vi "mqttCmdPublishCreate.vi"(6 "connMeta":T1, 8 "error in (no error)":errorcluster, 9 "value":string, 10 "topic":string) -> (0 "error out":errorcluster, 3 "mqttCmdPublish out":refnum<class "PublishMqttMsg.lvclass">)   [LabVIEW 2020, in "PublishMqttMsg.lvclass"]
uses:
  PublishMqttMsg.lvclass
  mqttTypedef/ConnectionMeta.ctl
  mqttTypedef/QosLevel.ctl
  PublishMqttMsg.lvclass/PublishMqttMsg.ctl
  BaseMqttMsg.lvclass
  MQTT Client.lvclass
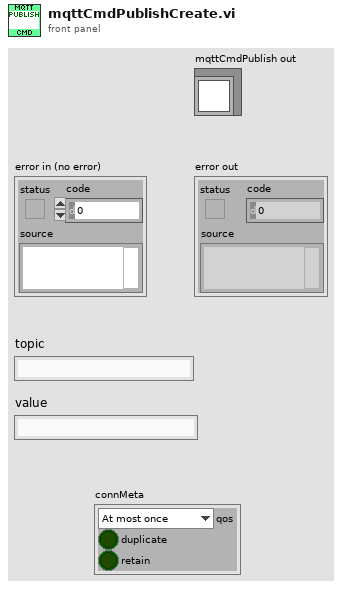
[diagram p1: front panel]
types:
  T1 = typedef "MQTT Client.lvclass/ConnectionMeta.ctl" = cluster{"qos":T2, "duplicate":bool, "retain":bool}
  T2 = typedef "BaseMqttMsg.lvclass/QosLevel.ctl" = enum8{"At most once", "At least once", "Exactly once", "Reserved"}
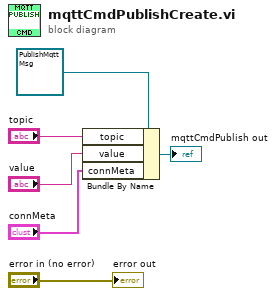
[diagram p0: block diagram]
diagram:
  n1 = Bundle By Name(cluster=refnum<class "PublishMqttMsg.lvclass"> refnum ("mqttCmdPublish in"), "topic"="topic", "value"="value", "connMeta"="connMeta") -> (→"mqttCmdPublish out":refnum<class "PublishMqttMsg.lvclass">)
  "error out" <- "error in (no error)"
